vi "3D Tracking Trajectory Helix Tracking Circle.vi"() -> ()   [LabVIEW 2018]
uses:
  <vilib>/Utility/file.llb/Read Delimited Spreadsheet (string).vi
  <vilib>/vision/NI_Vision_Development_Module.lvlib
panel:
  out "侧视range":cluster{"Replace Value":sgl, "a":dbl}
  in  "redwidth":u32=3
  in  "blackwidth":u32=2
  out "俯视range":cluster{"Replace Value":sgl, "a":dbl}
  out "侧视轨迹图":T1(plugin-control)
  out "Image 11":T1(plugin-control)
  out "i":i32[](array[numeric])
  out "侧视原图":T1(plugin-control)
  in  "轨迹打开":bool
  in  "Settings 2":T2={"Objects"=0, "Threshold"=128, "Reject Border"=FALSE, "Fill Holes"=FALSE, "Min Object Size"=TRUE, "Min Size"=30, "Max Object Size"=TRUE, "Max Size"=500, "Show Search Area"=FALSE, "Show Center"=TRUE, "Show Bounding Box"=TRUE} {"Objects" items=["Bright Objects", "Dark Objects"]; "Threshold" min=1 max=999999999 step=1; "Max Size" min=1 max=999999999 step=1; "Min Size" min=1 max=999999999 step=1}
  out "Objects 2":T3(array[cluster]) {"Aspect Ratio" format="%.2f"; "Orientation" format="%.2f"; "Area" format="%.2f"; "Object Center"."Y" format="%.2f"; "Object Center"."X" format="%.2f"}
  in  "AVI File Path 2":path=path "H:/0701单个避障修复/三角侧视2.avi"
  out "轨迹跟踪点数":i32
  out "c2":dbl
  out "z":dbl
  out "y":dbl
  out "x":dbl
  out "b2":dbl
  out "a2":dbl
  out "b":dbl[](array[numeric])
  in  "pp":dbl
  out "与目标点的距离":sgl
  in  "guiji":path=path "I:/0628星星2/helix主程序修改0518最新/small_myRIO_Helmholtz - 1111ke4/0627新的三角形.txt" caption="call7-8"
  out "i":i32
  in  "Settings":T2={"Objects"=0, "Threshold"=128, "Reject Border"=FALSE, "Fill Holes"=FALSE, "Min Object Size"=TRUE, "Min Size"=20, "Max Object Size"=TRUE, "Max Size"=500, "Show Search Area"=FALSE, "Show Center"=TRUE, "Show Bounding Box"=TRUE} {"Objects" items=["Bright Objects", "Dark Objects"]; "Threshold" min=1 max=999999999 step=1; "Max Size" min=1 max=999999999 step=1; "Min Size" min=1 max=999999999 step=1}
  out "俯视轨迹图":T1(plugin-control)
  out "Objects":T3(array[cluster]) {"Aspect Ratio" format="%.2f"; "Orientation" format="%.2f"; "Area" format="%.2f"; "Object Center"."Y" format="%.2f"; "Object Center"."X" format="%.2f"}
  in  "停止":bool
  in  "AVI File Path":path=path "H:/0701单个避障修复/三角俯视2.avi"
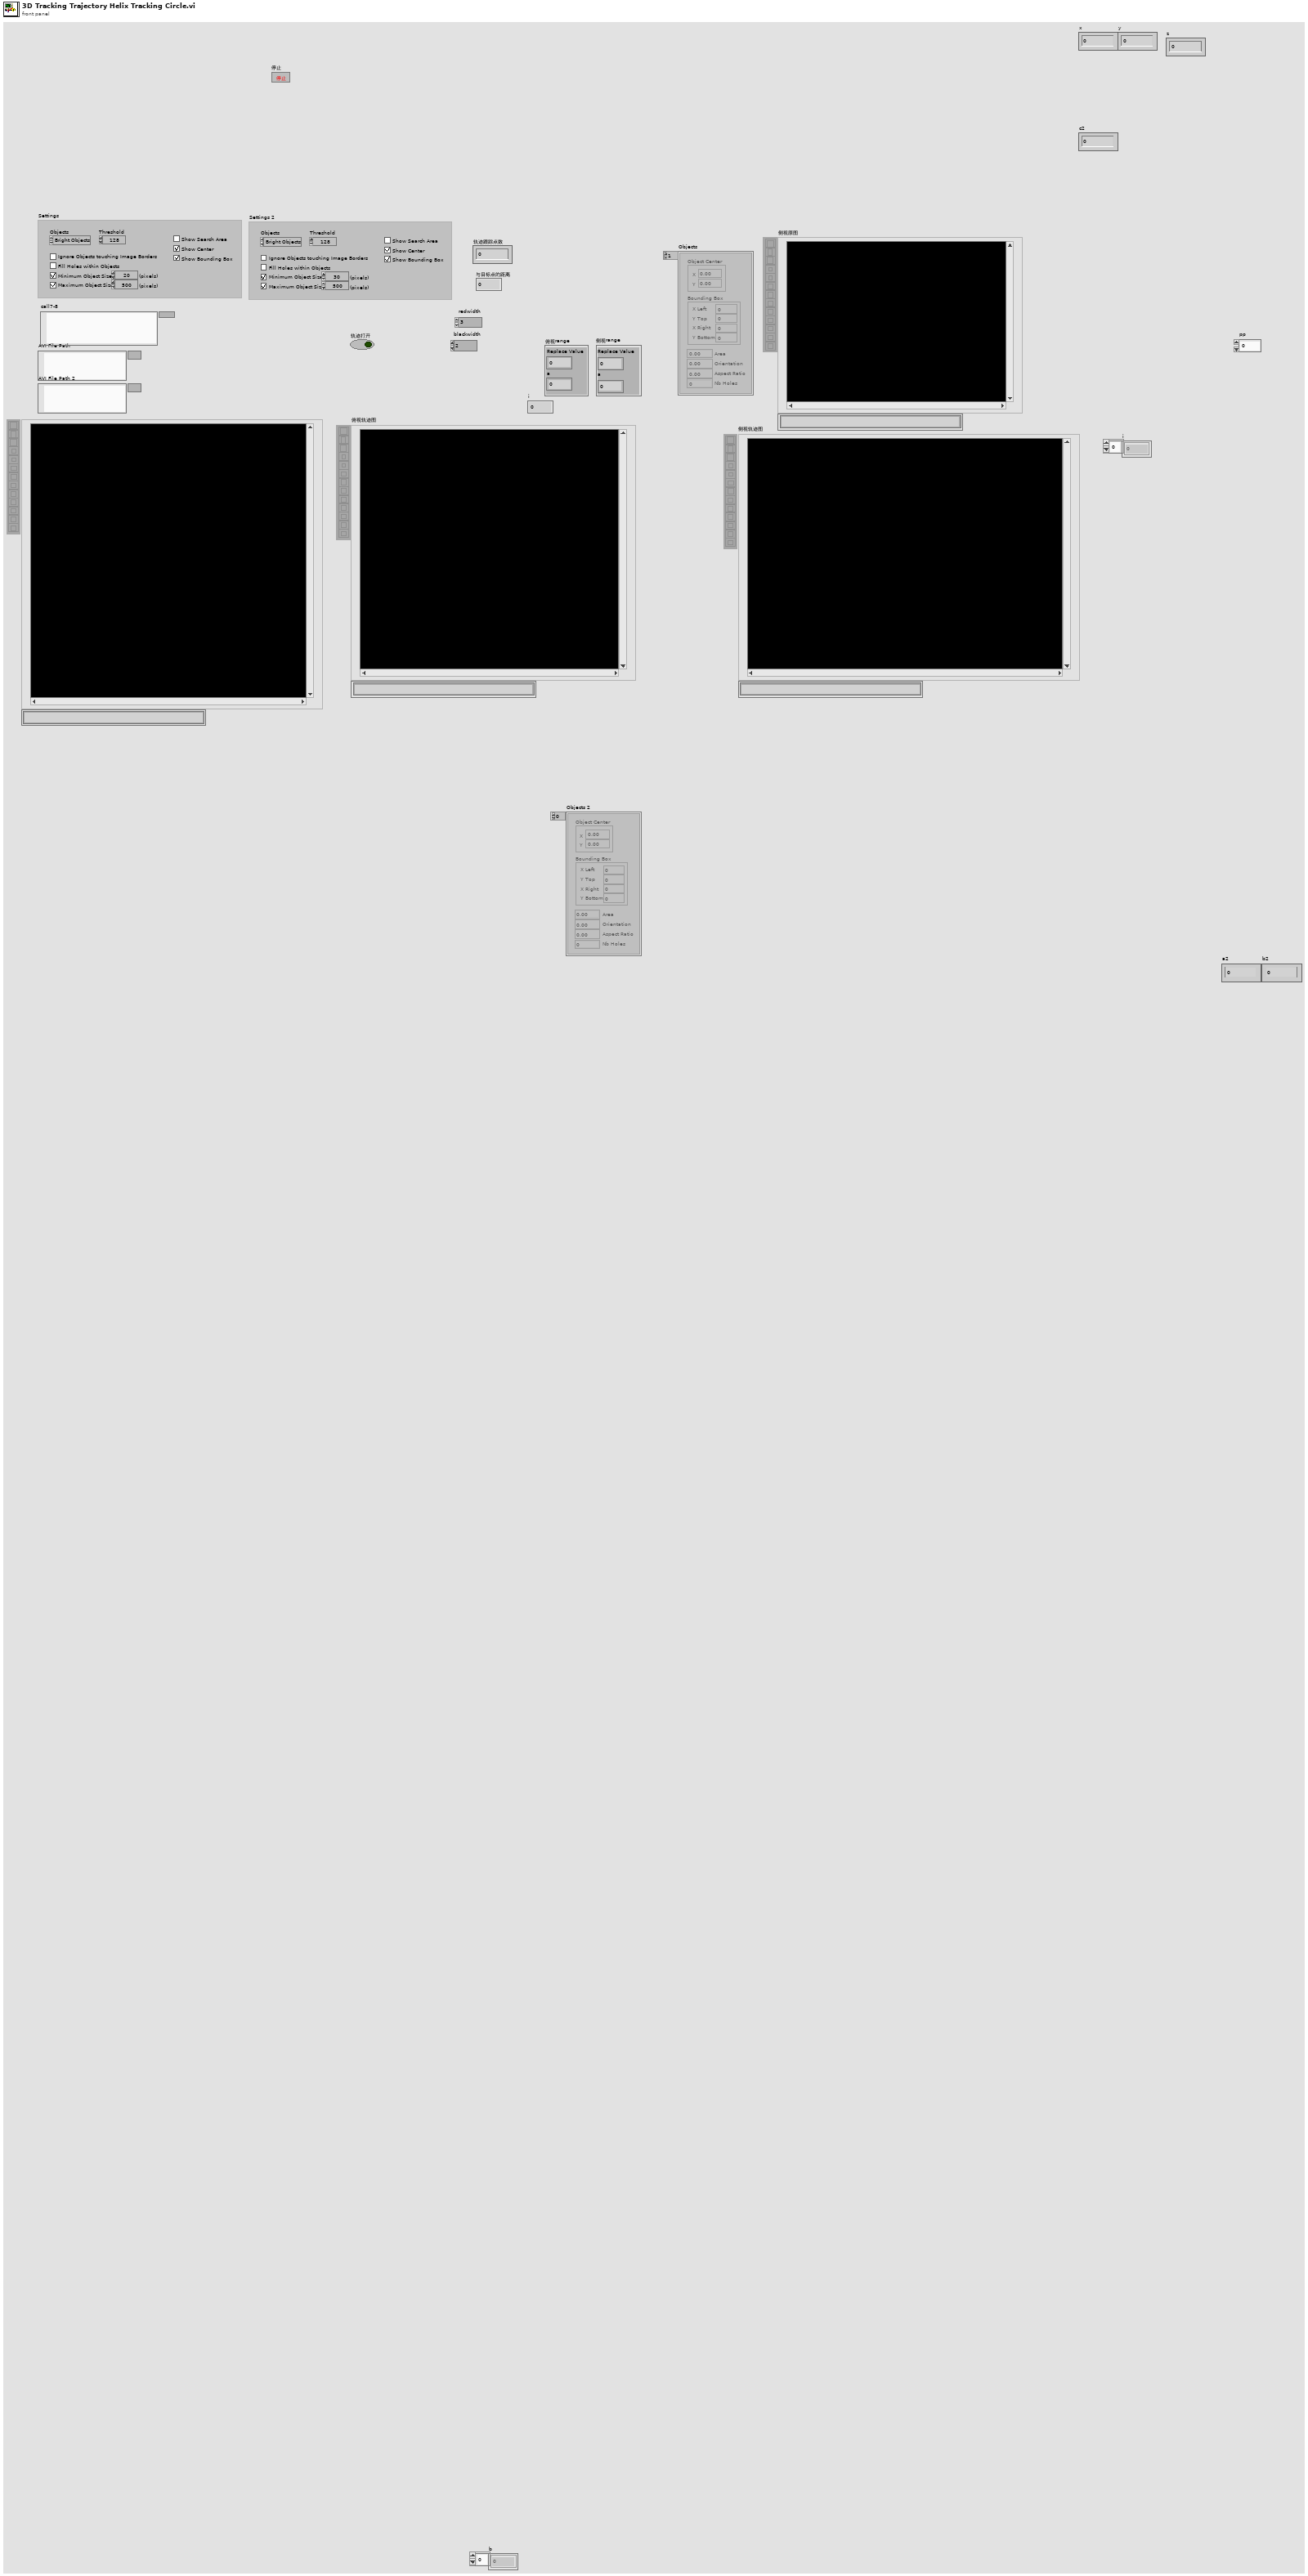
[diagram p1: front panel]
types:
  T1 = typedef "IMAQ Image.ctl" = refnum<image>
  T2 = cluster{"Objects":u16, "Threshold":i32, "Reject Border":bool, "Fill Holes":bool, "Min Object Size":bool, "Min Size":i32, "Max Object Size":bool, "Max Size":i32, "Show Search Area":bool, "Show Center":bool, "Show Bounding Box":bool}
  T3 = cluster{"Object Center":cluster{"X":sgl, "Y":sgl}, "Bounding Box":cluster{"X Left":i32, "Y Top":i32, "X Right":i32, "Y Bottom":i32}, "Area":sgl, "Orientation":sgl, "Aspect Ratio":sgl, "Nb Holes":i32}[]
  T4 = typedef "Image Type" = u32
  T5 = typedef "IMAQ AVI2 Refnum.ctl" = refnum<k20>
  T6 = cluster{"Objects[0]":cluster{"Object Center":cluster{"X":sgl, "Y":sgl}, "Bounding Box":cluster{"X Left":i32, "Y Top":i32, "X Right":i32, "Y Bottom":i32}, "Area":sgl, "Orientation":sgl, "Aspect Ratio":sgl, "Nb Holes":i32}, "Objects[1]":cluster{"Object Center":cluster{"X":sgl, "Y":sgl}, "Bounding Box":cluster{"X Left":i32, "Y Top":i32, "X Right":i32, "Y Bottom":i32}, "Area":sgl, "Orientation":sgl, "Aspect Ratio":sgl, "Nb Holes":i32}, "Objects[2]":cluster{"Object Center":cluster{"X":sgl, "Y":sgl}, "Bounding Box":cluster{"X Left":i32, "Y Top":i32, "X Right":i32, "Y Bottom":i32}, "Area":sgl, "Orientation":sgl, "Aspect Ratio":sgl, "Nb Holes":i32}, "Objects[3]":cluster{"Object Center":cluster{"X":sgl, "Y":sgl}, "Bounding Box":cluster{"X Left":i32, "Y Top":i32, "X Right":i32, "Y Bottom":i32}, "Area":sgl, "Orientation":sgl, "Aspect Ratio":sgl, "Nb Holes":i32}, "Objects[4]":cluster{"Object Center":cluster{"X":sgl, "Y":sgl}, "Bounding Box":cluster{"X Left":i32, "Y Top":i32, "X Right":i32, "Y Bottom":i32}, "Area":sgl, "Orientation":sgl, "Aspect Ratio":sgl, "Nb Holes":i32}, "Objects[5]":cluster{"Object Center":cluster{"X":sgl, "Y":sgl}, "Bounding Box":cluster{"X Left":i32, "Y Top":i32, "X Right":i32, "Y Bottom":i32}, "Area":sgl, "Orientation":sgl, "Aspect Ratio":sgl, "Nb Holes":i32}, "Objects[6]":cluster{"Object Center":cluster{"X":sgl, "Y":sgl}, "Bounding Box":cluster{"X Left":i32, "Y Top":i32, "X Right":i32, "Y Bottom":i32}, "Area":sgl, "Orientation":sgl, "Aspect Ratio":sgl, "Nb Holes":i32}, "Objects[7]":cluster{"Object Center":cluster{"X":sgl, "Y":sgl}, "Bounding Box":cluster{"X Left":i32, "Y Top":i32, "X Right":i32, "Y Bottom":i32}, "Area":sgl, "Orientation":sgl, "Aspect Ratio":sgl, "Nb Holes":i32}, "Objects[8]":cluster{"Object Center":cluster{"X":sgl, "Y":sgl}, "Bounding Box":cluster{"X Left":i32, "Y Top":i32, "X Right":i32, "Y Bottom":i32}, "Area":sgl, "Orientation":sgl, "Aspect Ratio":sgl, "Nb Holes":i32}}
  T7 = cluster{"Object Center":cluster{"X":sgl, "Y":sgl}, "Bounding Box":cluster{"X Left":i32, "Y Top":i32, "X Right":i32, "Y Bottom":i32}, "Area":sgl, "Orientation":sgl, "Aspect Ratio":sgl, "Nb Holes":i32}
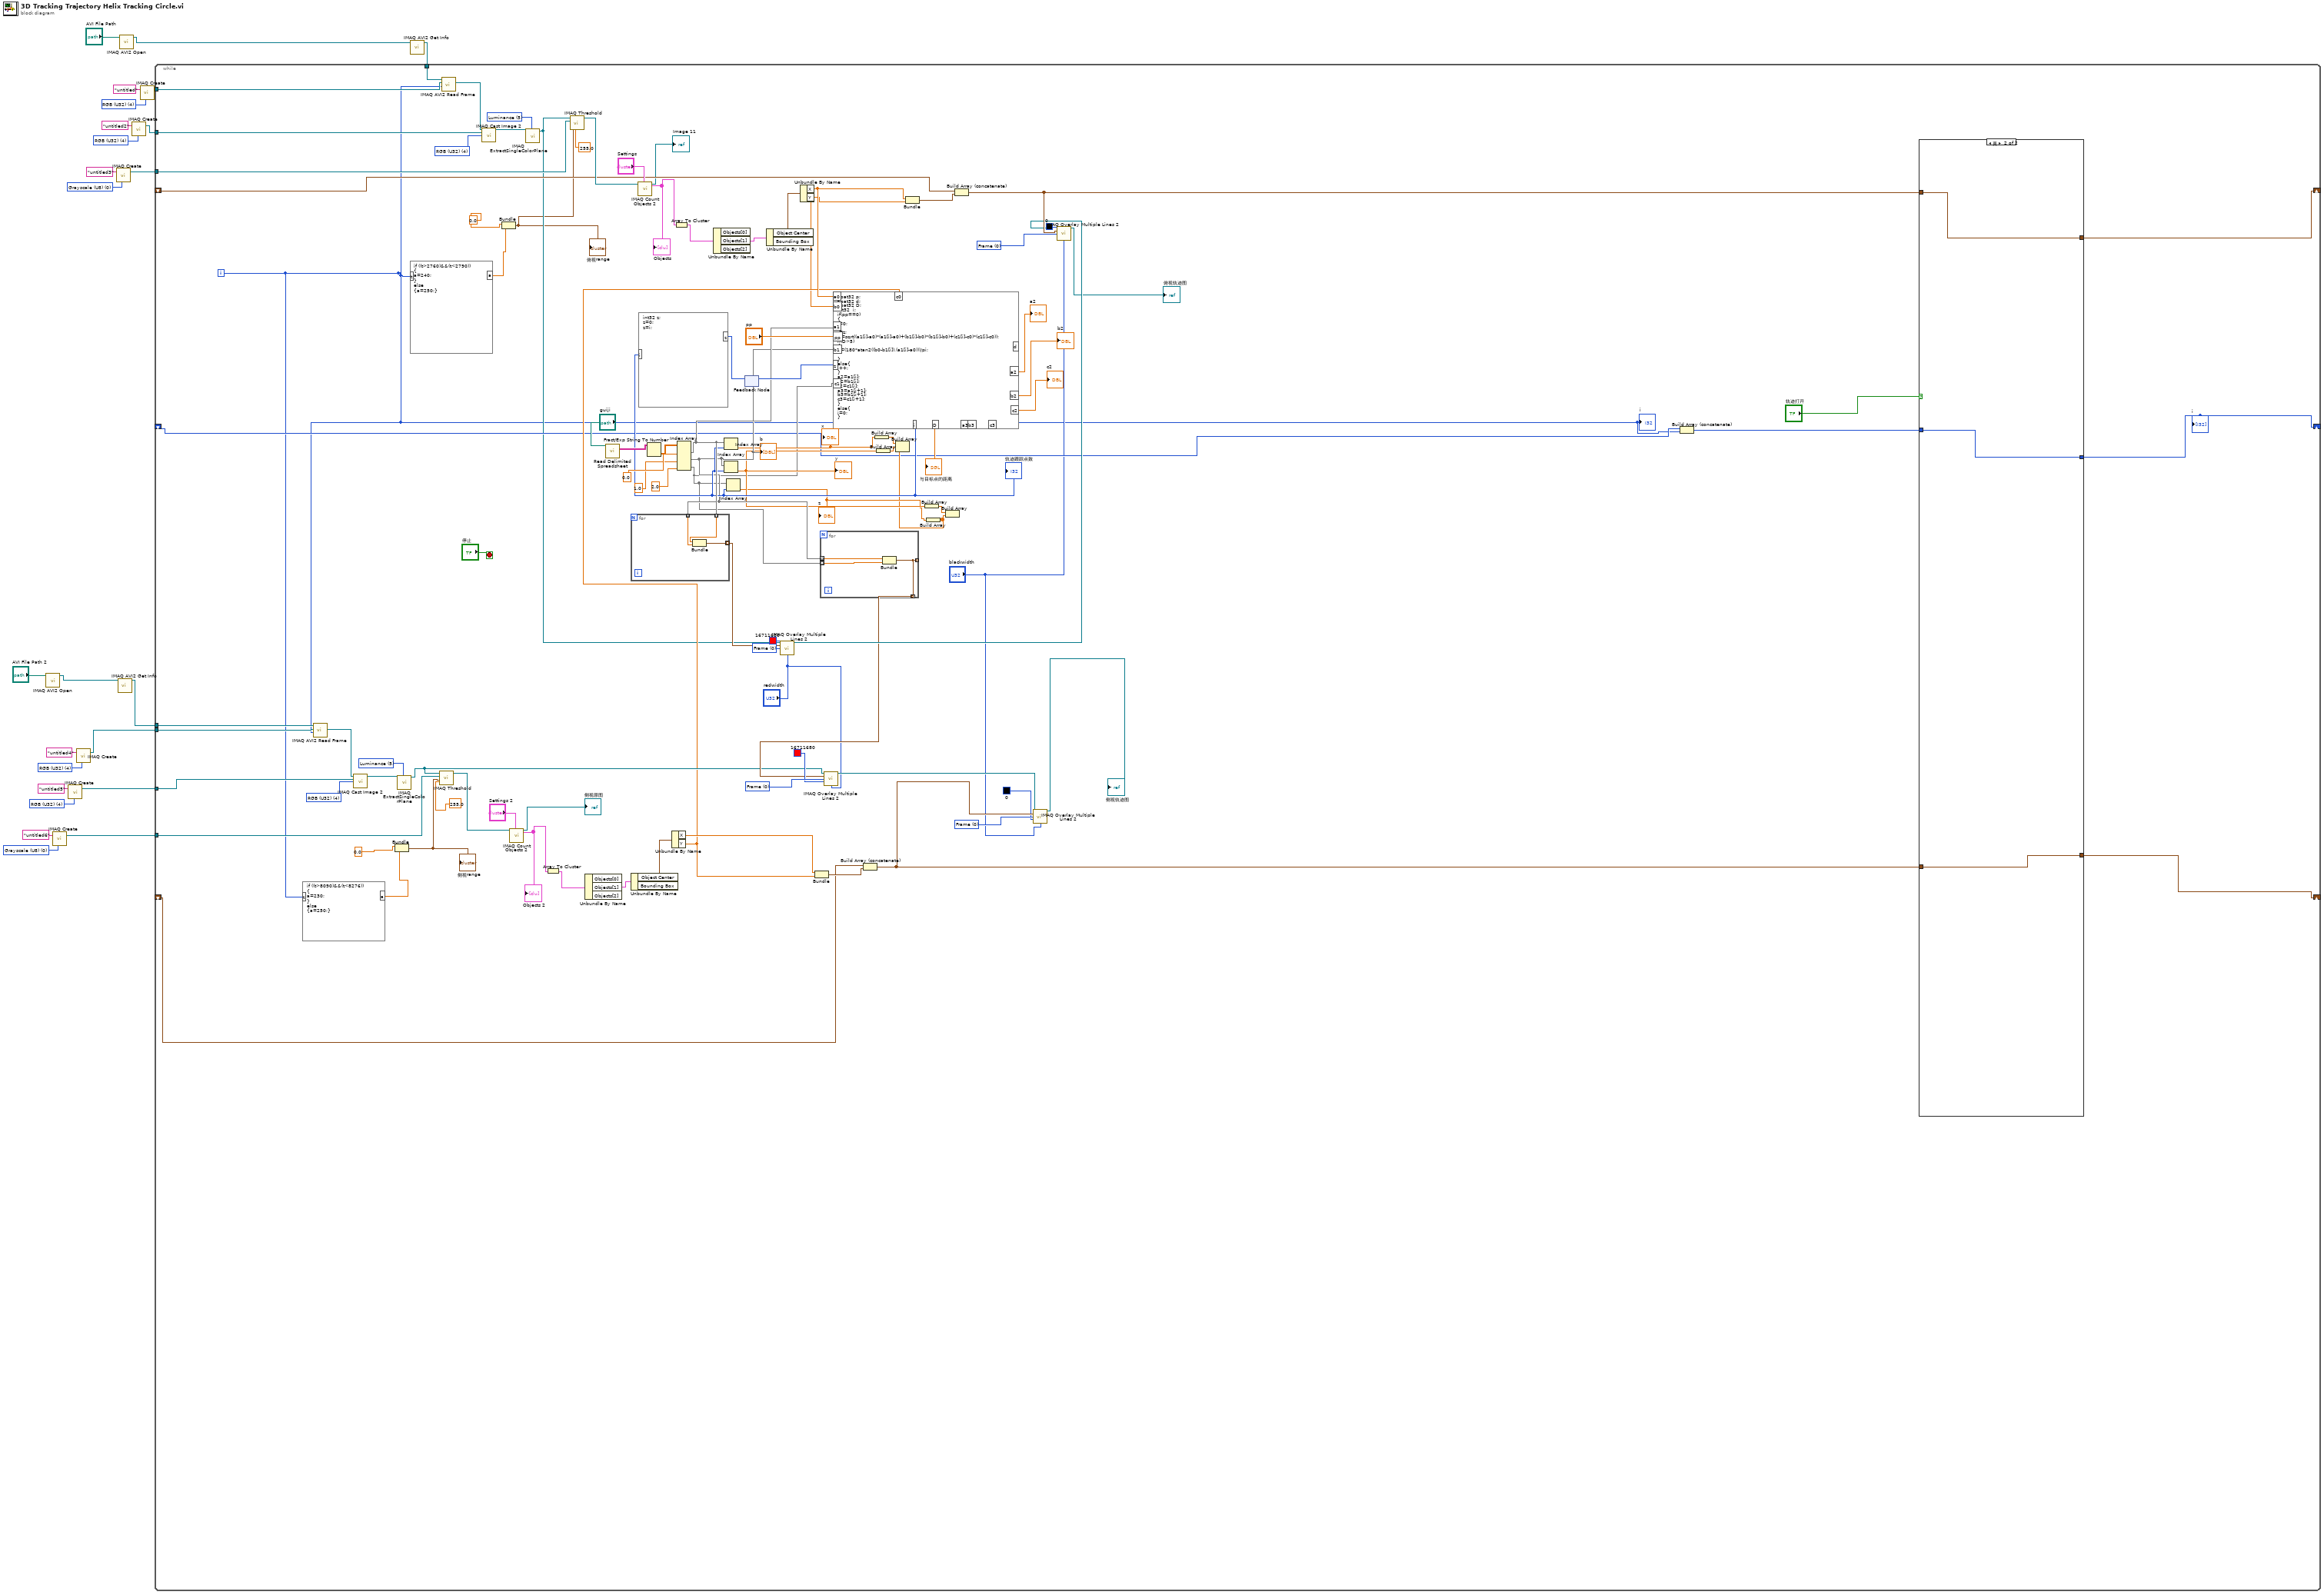
[diagram p0: block diagram]
diagram:
  w9 = T4 0 items=["Grayscale (U8)", "Grayscale (I16)", "Grayscale (SGL)", "Complex (CSG)", "RGB (U32)", "HSL (U32)", "RGB (U64)", "Grayscale (U16)"] ("Image Type")
  w7 = T4 4 items=["Grayscale (U8)", "Grayscale (I16)", "Grayscale (SGL)", "Complex (CSG)", "RGB (U32)", "HSL (U32)", "RGB (U64)", "Grayscale (U16)"] ("Image Type")
  w5 = T4 4 items=["Grayscale (U8)", "Grayscale (I16)", "Grayscale (SGL)", "Complex (CSG)", "RGB (U32)", "HSL (U32)", "RGB (U64)", "Grayscale (U16)"] ("Image Type")
  w17 = T4 0 items=["Grayscale (U8)", "Grayscale (I16)", "Grayscale (SGL)", "Complex (CSG)", "RGB (U32)", "HSL (U32)", "RGB (U64)", "Grayscale (U16)"] ("Image Type")
  w20 = T4 4 items=["Grayscale (U8)", "Grayscale (I16)", "Grayscale (SGL)", "Complex (CSG)", "RGB (U32)", "HSL (U32)", "RGB (U64)", "Grayscale (U16)"] ("Image Type")
  w22 = T4 4 items=["Grayscale (U8)", "Grayscale (I16)", "Grayscale (SGL)", "Complex (CSG)", "RGB (U32)", "HSL (U32)", "RGB (U64)", "Grayscale (U16)"] ("Image Type")
  n1 = call "IMAQ AVI2 Open"("AVI File Path"="AVI File Path 2") -> ("AVI Refnum"=w11:T5)  [unwired: 9 in, 1 out]
  n2 = call "IMAQ Create"("Image Name"="untitled6", "Image Type"=w9) -> ("New Image"=w2:T1)  [unwired: 3 in, 1 out]
  n3 = call "IMAQ Create"("Image Name"="untitled5", "Image Type"=w7) -> ("New Image"=w1:T1)  [unwired: 3 in, 1 out]
  n4 = call "IMAQ Create"("Image Name"="untitled4", "Image Type"=w5) -> ("New Image"=w3:T1)  [unwired: 3 in, 1 out]
  n5 = call "IMAQ Create"("Image Name"="untitled3", "Image Type"=w17) -> ("New Image"=w19:T1)  [unwired: 3 in, 1 out]
  n6 = call "IMAQ AVI2 Get Info"("AVI Refnum"=w11) -> ("AVI Refnum (duplicate)"=w4:T5)  [unwired: 6 in, 4 out]
  n7 = call "IMAQ AVI2 Open"("AVI File Path"="AVI File Path") -> ("AVI Refnum"=w14:T5)  [unwired: 9 in, 1 out]
  n8 = call "IMAQ Create"("Image Name"="untitled2", "Image Type"=w20) -> ("New Image"=w21:T1)  [unwired: 3 in, 1 out]
  n9 = call "IMAQ Create"("Image Name"="untitled", "Image Type"=w22) -> ("New Image"=w16:T1)  [unwired: 3 in, 1 out]
  n10 = call "IMAQ AVI2 Get Info"("AVI Refnum"=w14) -> ("AVI Refnum (duplicate)"=w13:T5)  [unwired: 6 in, 4 out]
  n11 = while {
    tunnel: w21 -> [w122]
    tunnel: w19 -> [w119]
    tunnel: w16 -> [w117]
    tunnel: w13 -> [w116]
    tunnel: w4 -> [w79]
    tunnel: w3 -> [w78]
    tunnel: w2 -> [w77]
    tunnel: w1 -> [w76]
    shift-right: [w66] -> _
    shift-left: _ -> [w65]
    shift-right: [w52] -> _
    shift-left: _ -> [w51]
    shift-right: [w43] -> _
    shift-left: _ -> [w41]
    i -> [w26]
    stop <- "停止" stop-if-true
    w50 = u32 0 items=["Frame", "Fill"] ("Drawing Mode (Frame)")
    w59 = u32 0 items=["Frame", "Fill"] ("Drawing Mode (Frame)")
    w64 = u32 0 items=["Frame", "Fill"] ("Drawing Mode (Frame)")
    w70 = u32 0 items=["Frame", "Fill"] ("Drawing Mode (Frame)")
    w87 = T4 4 items=["Grayscale (U8)", "Grayscale (I16)", "Grayscale (SGL)", "Complex (CSG)", "RGB (U32)", "HSL (U32)", "RGB (U64)", "Grayscale (U16)"] ("Image Type")
    w88 = 5 items=["Red", "Green", "Blue", "Hue", "Saturation", "Luminance", "Value", "Intensity"] ("Color Plane")
    w120 = T4 4 items=["Grayscale (U8)", "Grayscale (I16)", "Grayscale (SGL)", "Complex (CSG)", "RGB (U32)", "HSL (U32)", "RGB (U64)", "Grayscale (U16)"] ("Image Type")
    w121 = 5 items=["Red", "Green", "Blue", "Hue", "Saturation", "Luminance", "Value", "Intensity"] ("Color Plane")
    n12 = formula code="if ((t>8090)&&(t<8276))\n{\na=230;\n}\nelse\n{a=250;}"("t"=w26) -> ("a"=w27:dbl)
    n13 = call "IMAQ AVI2 Read Frame"("Frame Number"=w26, "Image"=w78, "AVI Refnum"=w79) -> ("Image Out"=w75:T1)  [unwired: 6 in, 2 out]
    n14 = call "IMAQ Cast Image 2"("Image Src"=w75, "Image Dst"=w76, "Image Type"=w87) -> ("Image Dst Out"=w83:T1)  [unwired: 11 in, 1 out]
    n15 = Bundle("Replace Value"=sgl 0.0, "a"=w27) -> (w25:cluster{"Replace Value":sgl, "a":dbl})  [unwired: 1 in]
    "侧视range" <- w25
    n16 = call "IMAQ ExtractSingleColorPlane"("Color Plane"=w88, "Image Src"=w83) -> ("Image Dst Out"=w56:T1)  [unwired: 8 in, 1 out]
    n17 = formula code="if ((t>2760)&&(t<2790))\n{\na=240;\n}\nelse\n{a=250;}"("t"=w26) -> ("a"=w33:dbl)
    n18 = call "IMAQ Threshold"("Replace Value"=sgl 255.0, "Range"=w25, "Image Dst"=w77, "Image Src"=w56) -> ("Image Dst Out"=w81:T1)  [unwired: 6 in, 1 out]
    n19 = call "IMAQ AVI2 Read Frame"("Frame Number"=w26, "Image"=w117, "AVI Refnum"=w116) -> ("Image Out"=w40:T1)  [unwired: 6 in, 2 out]
    n20 = call "IMAQ Cast Image 2"("Image Src"=w40, "Image Dst"=w122, "Image Type"=w120) -> ("Image Dst Out"=w113:T1)  [unwired: 11 in, 1 out]
    n21 = Bundle("Replace Value"=sgl 0.0, "a"=w33) -> (w31:cluster{"Replace Value":sgl, "a":dbl})  [unwired: 1 in]
    "俯视range" <- w31
    n22 = call "IMAQ Count Objects 2"("Settings"="Settings 2", "Image"=w81) -> ("Image Out"=→"侧视原图":T1, "Objects"=w85:T3)  [unwired: 5 in, 3 out]
    "Objects 2" <- w85
    n23 = call "IMAQ ExtractSingleColorPlane"("Color Plane"=w121, "Image Src"=w113) -> ("Image Dst Out"=w39:T1)  [unwired: 8 in, 1 out]
    n24 = Array To Cluster(array=w85) -> (cluster=w84:T6)
    n25 = call "IMAQ Threshold"("Replace Value"=sgl 255.0, "Range"=w31, "Image Dst"=w119, "Image Src"=w39) -> ("Image Dst Out"=w111:T1)  [unwired: 6 in, 1 out]
    n26 = Unbundle By Name(w84) -> ("Objects[1]"=w36:T7)  [unwired: 2 out]
    n27 = call-poly <vilib>:"Read Delimited Spreadsheet.vi"("file path (dialog if empty)"="guiji") -> ("all rows"=w108:string[][])  [unwired: 9 in, 5 out]
    n28 = Unbundle By Name(w36) -> ("Object Center"=w80:cluster{"X":sgl, "Y":sgl})  [unwired: 1 out]
    n29 = call "IMAQ Count Objects 2"("Settings"="Settings", "Image"=w111) -> ("Image Out"=→"Image 11":T1, "Objects"=w114:T3)  [unwired: 5 in, 3 out]
    "Objects" <- w114
    n30 = Fract/Exp String To Number(string=w108) -> (number=w107:dbl[][])  [unwired: 3 in, 1 out]
    n31 = Unbundle By Name(w80) -> ("X"=w54:sgl, "Y"=w53:sgl)
    n32 = Array To Cluster(array=w114) -> (cluster=w35:T6)
    n33 = Index Array(array=w107, index (col) #1=0.0, index (col) #2=1.0, index (col) #3=2.0) -> (element #1=w100:dbl[], element #2=w97:dbl[], element #3=w90:dbl[])  [unwired: 3 in]
    "b" <- w97
    n34 = for {
      tunnel: w100 -> [w131] mode=indexing
      tunnel: w97 -> [w130] mode=indexing
      tunnel: [w129] -> w71 mode=indexing
      n35 = Bundle("String"=w131, "String"=w130) -> (w129:cluster{"String":dbl, "String":dbl})  [unwired: 1 in]
    }
    n36 = Unbundle By Name(w35) -> ("Objects[1]"=w32:T7)  [unwired: 2 out]
    n37 = feedback #1() -> (w103:i32)  [unwired: 1 in]
    n38 = Unbundle By Name(w32) -> ("Object Center"=w110:cluster{"X":sgl, "Y":sgl})  [unwired: 1 out]
    n39 = call "IMAQ Overlay Multiple Lines 2"("Image"=w39, "Line End Points"=w71, "Drawing Mode (Frame)"=w70, "Color"=u32 16711680, "Width"="redwidth") -> ("Image Out"=w61:T1)  [unwired: 9 in, 1 out]
    n40 = Unbundle By Name(w110) -> ("X"=w68:sgl, "Y"=w45:sgl)
    n41 = Bundle("X"=w54, "Y"=w53) -> (w55:cluster{"X":sgl, "Y":sgl})  [unwired: 1 in]
    n42 = for {
      tunnel: [w126] -> _ mode=indexing
      tunnel: w97 -> [w128] mode=indexing
      tunnel: w90 -> [w127] mode=indexing
      tunnel: [w126] -> w57 mode=indexing
      n43 = Bundle("String"=w128, "String"=w127) -> (w126:cluster{"String":dbl, "String":dbl})  [unwired: 1 in]
    }
    n44 = call "IMAQ Overlay Multiple Lines 2"("Image"=w56, "Line End Points"=w57, "Drawing Mode (Frame)"=w59, "Color"=u32 16711680, "Width"="redwidth") -> ("Image Out"=w47:T1)  [unwired: 9 in, 1 out]
    n45 = formula code="float32 p;\nfloat32 d;\nfloat32 D;\nint32  i;\nif(pp==0)\n{\ni=0;\n\ni=z;\nD=sqrt((a1[i]-a0)*(a1[i]-a0)+(b1[i]-b0)*(b1[i]-b0)+(c1[i]-c0)*(c1[i]-c0));\nif(D>5)\n{\nd=(180*atan2((b0-b1[i]),(a1[i]-a0)))/pi;\n\n}\nelse{\ni++;\n}\na2=a1[i];\nb2=b1[i];\nc2=c1[i];\na3=a1[i+1];\nb3=b1[i+1];\nc3=c1[i+1];\n}\nelse{\ni=0;\n}"("a0"=w68, "b0"=w45, "a1"=w100, "b1"=w97, "z"=w103, "pp"="pp", "c1"=w90, "c0"=w53) -> ("i"=w98:i32, "D"=→"与目标点的距离":sgl, "a2"=→"a2":dbl, "b2"=→"b2":dbl, "c2"=→"c2":dbl)  [unwired: 4 out]
    "轨迹跟踪点数" <- w98
    n46 = formula code="int32 z;\nz=0;\nz=i;"("i"=w98) -> ("z"=w104:i32)
    n47 = Index Array(array=w100, index=w98) -> (element=w96:dbl)
    "x" <- w96
    n48 = Index Array(array=w97, index=w98) -> (element=w93:dbl)
    "y" <- w93
    n49 = Index Array(array=w90, index=w98) -> (element=w92:dbl)
    "z" <- w92
    n50 = feedback-in #1(w104) -> ()
    n51 = Build Array (concatenate)(w51, w55) -> (w49:cluster{"X":sgl, "Y":sgl}[])
    n52 = Build Array(w96) -> (w95:dbl[])
    n53 = Build Array(w93) -> (w94:dbl[])
    n54 = Bundle("X"=w68, "Y"=w45) -> (w67:cluster{"X":sgl, "Y":sgl})  [unwired: 1 in]
    n55 = Build Array(w93) -> (w91:dbl[])
    n56 = Build Array(w92) -> (w89:dbl[])
    n57 = Build Array(w95, w94, w89) -> ()  [unwired: 1 out]
    n58 = Build Array(w91, w89) -> ()  [unwired: 1 out]
    n59 = Build Array (concatenate)(w65, w67) -> (w62:cluster{"X":sgl, "Y":sgl}[])
    n60 = call "IMAQ Overlay Multiple Lines 2"("Image"=w47, "Line End Points"=w49, "Drawing Mode (Frame)"=w50, "Color"=u32 0, "Width"="blackwidth") -> ("Image Out"=→"侧视轨迹图":T1)  [unwired: 9 in, 1 out]
    n61 = call "IMAQ Overlay Multiple Lines 2"("Image"=w61, "Line End Points"=w62, "Drawing Mode (Frame)"=w64, "Color"=u32 0, "Width"="blackwidth") -> ("Image Out"=→"俯视轨迹图":T1)  [unwired: 9 in, 1 out]
    n62 = Build Array (concatenate)(w41, w26) -> (w42:i32[])
    n63 = case shown="真" "轨迹打开" {
      tunnel: [_ w125] -> w66
      tunnel: w62 -> [_ w125]
      tunnel: [_ w124] -> w52
      tunnel: w49 -> [_ w124]
      tunnel: [_ w123] -> w43
      tunnel: w42 -> [_ w123]
      frame False {
      }
      frame True {
      }
    }
    "i" <- w43
    "i" <- w26
  }
